vi "Nattify - Get BD Canvas Margin.vi"(11 "error in":errorcluster) -> (4 "BD canvas margin":i16, 15 "error out":errorcluster)   [LabVIEW 2020]
uses:
  <resource>/dialog/lvconfig.llb/LV Config Read Numeric (I32).vi
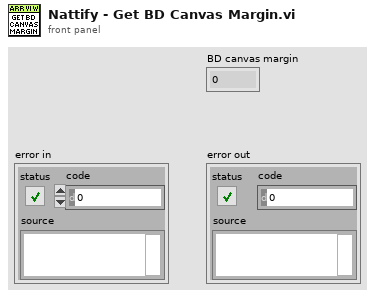
[diagram p1: front panel]
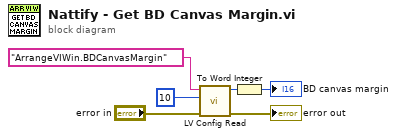
[diagram p0: block diagram]
diagram:
  n1 = call-poly <resource>:"LV Config Read.vi"("error in"="error in", "default value"=10, "key"="ArrangeVIWin.BDCanvasMargin" ("string")) -> ("error out"=→"error out":errorcluster, "value"=w3:i32)  [unwired: 2 in, 1 out]
  n2 = To Word Integer(number=w3) -> (16bit integer=→"BD canvas margin":i16)
